vi "Initialize-status-notifs.vi"(8 "error in (no error)":errorcluster, 11 "Object ref in":T1) -> (0 "error out":errorcluster, 3 "Object ref out":T1)   [LabVIEW 2013, in "PowderDeposition.lvlib" / "PD-Main.lvclass"]
uses:
  PD-Main.lvclass
  Object-reference.ctl
  PD-Main.lvclass/PD-Main.ctl
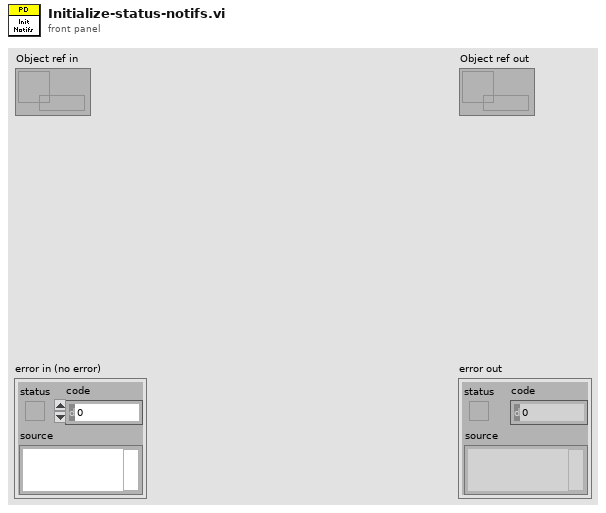
[diagram p1: front panel]
types:
  T1 = typedef "PowderDeposition.lvlib/PD-Main.lvclass/Object-reference.ctl" = refnum<data-value>
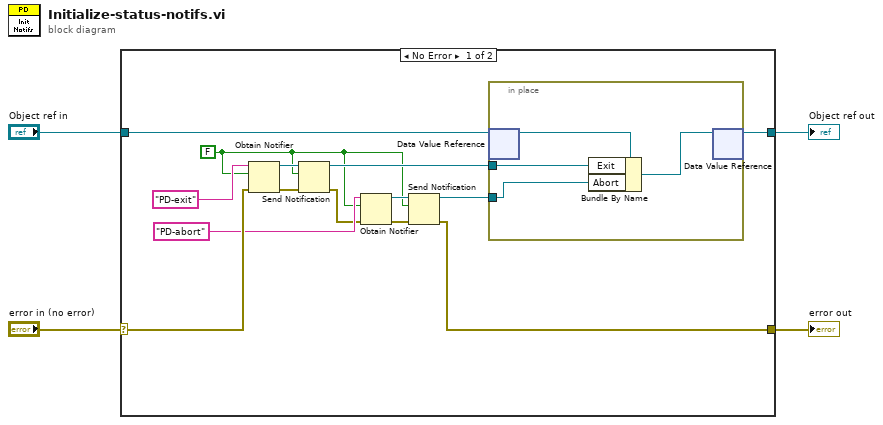
[diagram p0: block diagram]
diagram:
  n1 = case shown="No Error" "error in (no error)" {
    selector: "error in (no error)" -> [w15 w24]
    tunnel: [w6 w24] -> w3
    tunnel: [w17 w23] -> w1
    tunnel: "Object ref in" -> [w18 w23]
    frame No Error {
      w8 = FALSE
      n2 = Obtain Notifier(name (unnamed)="PD-exit", notification data type=w8, error in (no error)=w15) -> (notifier out=w16:refnum<notifier>, error out=w10:errorcluster)  [unwired: 1 in, 1 out]
      n3 = Send Notification(notification=w8, notifier=w16, error in (no error)=w10) -> (notifier out=w11:refnum<notifier>, error out=w5:errorcluster)
      n4 = Obtain Notifier(name (unnamed)="PD-abort", notification data type=w8, error in (no error)=w5) -> (notifier out=w14:refnum<notifier>, error out=w7:errorcluster)  [unwired: 1 in, 1 out]
      n5 = Send Notification(notification=w8, notifier=w14, error in (no error)=w7) -> (notifier out=w9:refnum<notifier>, error out=w6:errorcluster)
      n6 = in-place {
        in-place-border: w11 -> [w20]
        in-place-border: w9 -> [w19]
        n7 = in-place-dvr #1(w18) -> (w22:refnum<class "PD-Main.lvclass">)  [unwired: 1 out]
        n8 = Bundle By Name(cluster=w22, "Exit"=w20, "Abort"=w19) -> (w21:refnum<class "PD-Main.lvclass">)
        n9 = in-place-dvr #1(w21) -> (w17:T1)  [unwired: 1 out]
      }
    }
    frame Error {
    }
  }
  "error out" <- w3
  "Object ref out" <- w1
